vi "OpenVI.vi"(0 "name or relative path":string, 1 "stripped path":path) -> ()   [LabVIEW 2011]
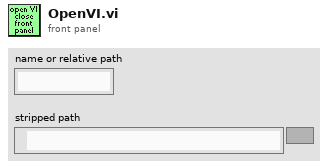
[diagram p1: front panel]
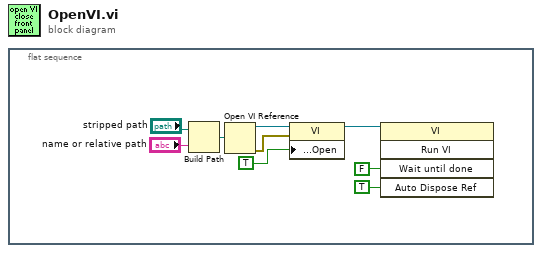
[diagram p0: block diagram]
diagram:
  n1 = flat-sequence {
    frame #0 {
      n2 = Build Path(base path="stripped path", name or relative path="name or relative path") -> (appended path=w4:path)
      n3 = Open VI Reference(vi path=w4) -> (vi reference=w1:refnum<vi>, error out=w7:errorcluster)  [unwired: 5 in]
      n4 = property class="VI"(reference=w1, error in=w7, "Front Panel.Open"=TRUE ("Auto Dispose Reference")) -> (reference out=w2:refnum<vi>)  [unwired: 1 out]
      n5 = invoke class="VI" method="Run VI"(reference=w2, "Wait until done"=FALSE ("Wait Until Done"), "Auto Dispose Ref"=TRUE ("Auto Dispose Reference")) -> ()  [unwired: 2 in, 5 out]
    }
  }
